vi "thcd_set_flt.vi"(5 "thcd_delay":u32=500, 6 "err_in":errorcluster, 7 "thcd_val":T1, 8 "thcd_ch":T2, 9 "thcd_visa":refnum<visa-resource-name>) -> (0 "err_out":errorcluster, 1 "thcd_st":bool, 2 "thcd_res_msg":string, 3 "thcd_visa":refnum<visa-resource-name>)   [LabVIEW 2018, in "1039_mod.lvlib"]
uses:
  thcd_controls/ctrl_chn_thcd.ctl
  thcd_controls/ctrl_flt_thcd.ctl
  1039_mod/1039_mod.lvlib
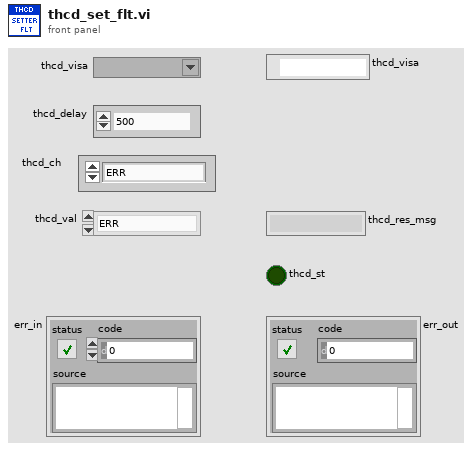
[diagram p1: front panel]
types:
  T1 = typedef "ctrl_flt_thcd.ctl" = enum16{"ERR", "4Hz", "15Hz", "30Hz", "100Hz"}
  T2 = typedef "ctrl_chn_thcd.ctl" = enum8{"ERR", "1", "2", "3", "4"}
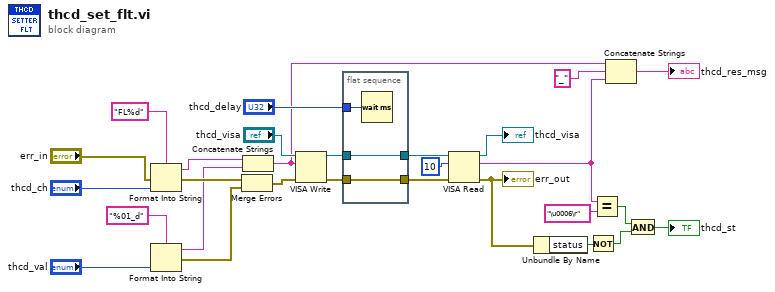
[diagram p0: block diagram]
diagram:
  n1 = Format Into String(format string="FL%d", error in="err_in", "thcd_ch") -> (resulting string=w20:string, error out=w19:errorcluster)  [unwired: 1 in]
  n2 = Format Into String(format string="%01_d", "thcd_val") -> (resulting string=w16:string, error out=w17:errorcluster)  [unwired: 2 in]
  n3 = Merge Errors(w19, w17) -> (w18:errorcluster)
  n4 = Concatenate Strings(w20, w16) -> (w2:string)
  n5 = VISA Write(VISA resource name="thcd_visa", write buffer=w2, error in (no error)=w18) -> (VISA resource name out=w27:refnum<visa-resource-name>, error out=w28:errorcluster)  [unwired: 1 out]
  n6 = flat-sequence {
    tunnel: w28 -> [w30]
    tunnel: [w30] -> w6
    tunnel: w27 -> [w29]
    tunnel: [w29] -> w7
    tunnel: "thcd_delay" -> [w31]
    frame #0 {
      n7 = Wait (ms)(milliseconds to wait=w31) -> ()  [unwired: 1 out]
    }
  }
  n8 = VISA Read(VISA resource name=w7, byte count=u32 10, error in (no error)=w6) -> (VISA resource name out=→"thcd_visa":refnum<visa-resource-name>, read buffer=w8:string, error out=w5:errorcluster)  [unwired: 1 out]
  "err_out" <- w5
  n9 = Unbundle By Name(w5) -> ("status"=w14:bool)
  n10 = Not(x=w14) -> (.not. x?=w11:bool)
  n11 = Equal?(x=w8, y="\u0006\r") -> (x = y?=w12:bool)
  n12 = Concatenate Strings(w2, "_", w8) -> (→"thcd_res_msg":string)
  n13 = And(x=w12, y=w11) -> (x .and. y?=→"thcd_st":bool)
